vi "QIandIQ_to_ComplexSample.vi"(8 "array size (samples)":i32=15, 10 "IQ or QI":bool=TRUE, 11 "Raw Data (Q,I) - base 10":T1) -> (0 "array size (samples)":i32, 2 "Complex Out":cdb[][](array[numeric]))   [LabVIEW 2016]
uses:
  <vilib>/Analysis/Matrix/Datatypes/RealMatrix.ctl
  <vilib>/Analysis/Matrix/Numeric/Complex/Cartesian To Complex - RM,RM.vi
  <vilib>/Analysis/Matrix/Numeric/Conversions/Matrix To Array - CM.vi
  <vilib>/Analysis/Matrix/NI_Matrix.lvlib
  <vilib>/Analysis/Matrix/Numeric/Conversions/Matrix To Array - RM.vi
panel:
  out "Raw Data (I) - base 10":T1
  out "Raw Data (Q) - base 10":T1
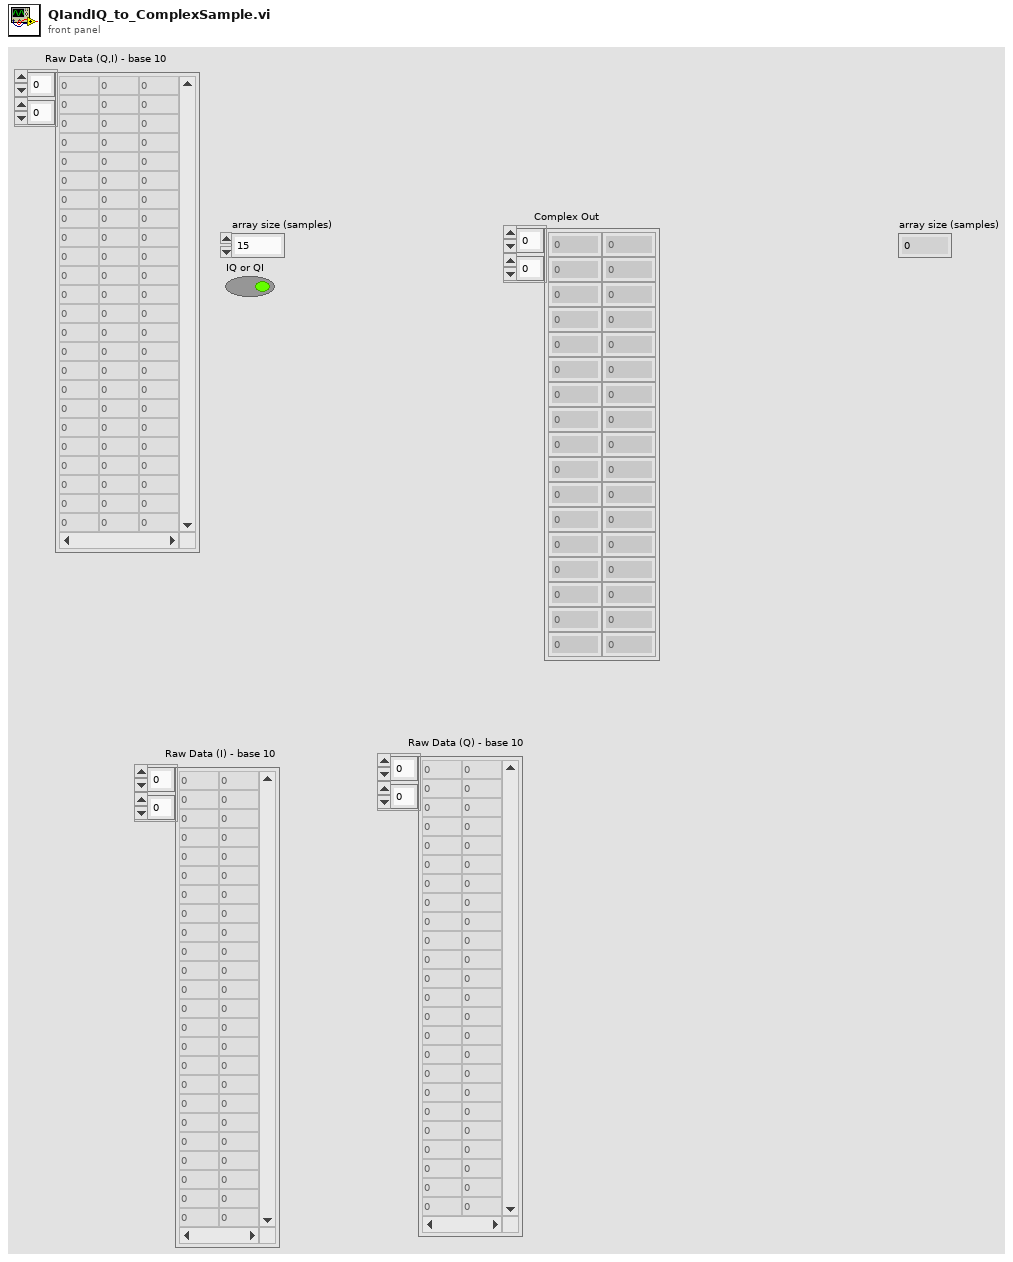
[diagram p1: front panel]
types:
  T1 = typedef "NI_Matrix.lvlib/RealMatrix.ctl" = dbl[][]
  T2 = typedef "NI_Matrix.lvlib/ComplexMatrix.ctl" = cdb[][]
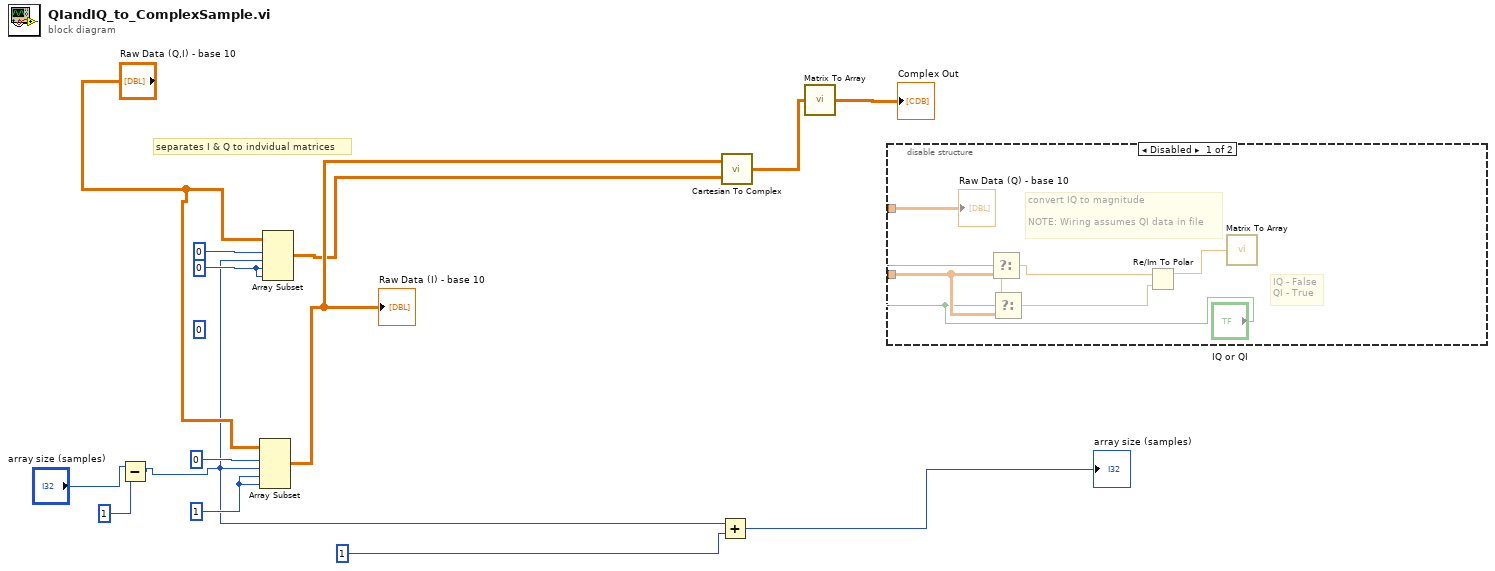
[diagram p0: block diagram]
diagram:
  w10 = 1 ("column N")
  (unwired) 0 ("column N")
  w9 = 0 ("column 1")
  # "separates I & Q to indvidual matrices"
  n1 = Subtract(x="array size (samples)", y=1) -> (x-y=w7:i32)
  n2 = Array Subset(array="Raw Data (Q,I) - base 10", index (row)=0 ("row 1"), length (row)=w7, index (col)=w10, length (col)=w10) -> (w4:T1)
  "Raw Data (I) - base 10" <- w4
  n3 = Array Subset(array="Raw Data (Q,I) - base 10", index (row)=0 ("row 1"), length (row)=w7, index (col)=w9, length (col)=w9) -> (w3:T1)
  n4 = Add(x=w7, y=1) -> (x+y=→"array size (samples)":i32)
  n5 = call-poly <vilib>:"Cartesian To Complex.vi"("Real Matrix I"=w3, "Real Matrix R"=w4) -> ("R + Ii"=w2:T2)
  n6 = call-poly <vilib>:"Matrix To Array.vi"("Complex Matrix"=w2) -> ("Complex 2D Array"=→"Complex Out":cdb[][])
  n7 = disable-structure shown="Disabled" {
    disable-tunnel: _ -> [w18 _]
    disable-tunnel: _ -> [w17 _]
    frame Disabled {
      # "IQ - False\nQI - True"
      # "convert IQ to magnitude\n\nNOTE: Wiring assumes QI data in file"
      n8 = Select(s="IQ or QI", f=w18) -> (t=w16:dbl, s? t:f=w19:dbl)
      n9 = Select(t=w16, s="IQ or QI", f=w18) -> (s? t:f=w20:dbl)
      n10 = Re/Im To Polar(2:w20, 3:w19) -> (1:w22:dbl)  [unwired: 1 out]
      n11 = call-poly <vilib>:"Matrix To Array.vi"("Real Matrix"=w22) -> ("Real 2D Array"=w21:dbl[][])
      "Raw Data (Q) - base 10" <- w17
    }
    frame Enabled {
    }
  }
